vi "ReportOUT.vi"(0 "Full/Fails":string(combo)="Full", 1 "Operator":string, 2 "Original ATR Ref":refnum<vi>, 3 "GeneralResult":bool, 4 "Header Array":string[][](array[string]), 5 "error in (no error)":errorcluster, 6 "Header":string="                          Searcher EPC/Micro Card ATR", 7 "report file path":path, 8 "PN":string) -> (19 "error out":errorcluster)   [LabVIEW 2017]
uses:
  <vilib>/Utility/miscctls.llb/LVRowAndColumnUnsignedTypeDef.ctl
  <vilib>/Utility/NIReport.llb/Append Image to Report (path wrap).vi
  <vilib>/Utility/NIReport.llb/Append Text Table to Report (wrap).vi
  <vilib>/Utility/NIReport.llb/Append Report Text (str wrap).vi
  <vilib>/Utility/NIReport.llb/NI_report.lvclass
  <vilib>/Utility/NIReport.llb/Word/NI_Word.lvclass
  <vilib>/addons/_office/NI_ReportGenerationToolkit.lvlib
panel:
  in  "Pass  Button":bool
  in  "Fail  Button":bool
  in  "ATR To .docx":string[][](table)=array1670x7[11690 elements] caption="ATR"
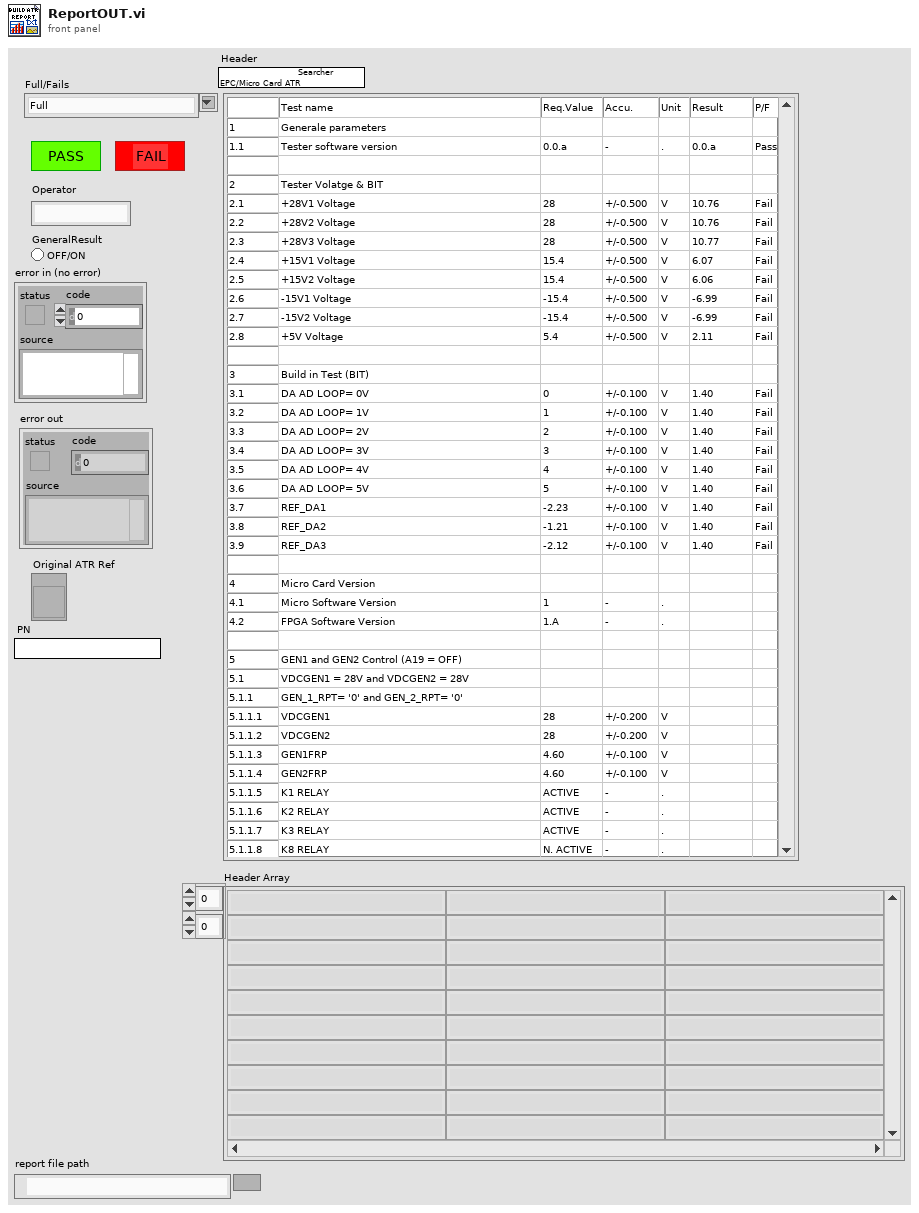
[diagram p1: front panel]
types:
  T1 = cluster{"top":dbl, "left":dbl, "right":dbl, "bottom":dbl}
  T2 = cluster{"alignment":enum16{"Left", "Centered", "Right", "Justify"}, "left":dbl, "right":dbl, "special":enum16{"(none)", "First line", "Hanging"}, "by":dbl, "before":dbl, "after":dbl, "line spacing":enum16{"Single", "1,5 lines", "Double", "At least", "Exactly", "Multiple"}, "at":dbl}
  T3 = enum16{"maximized", "minimized", "normal", "no change"}
  T4 = enum16{"Standard Report", "HTML", "Word", "Excel"}
  T5 = typedef "LVRowAndColumnUnsignedTypeDef.ctl" = cluster{"Row":u32, "Column":u32}
  T6 = typedef "LVFontTypeDef.ctl" = cluster{"Font Name":string, "Size":u16, "Bold":bool, "Italic":bool, "Underline":bool, "Strikeout":bool, "Color":u32}
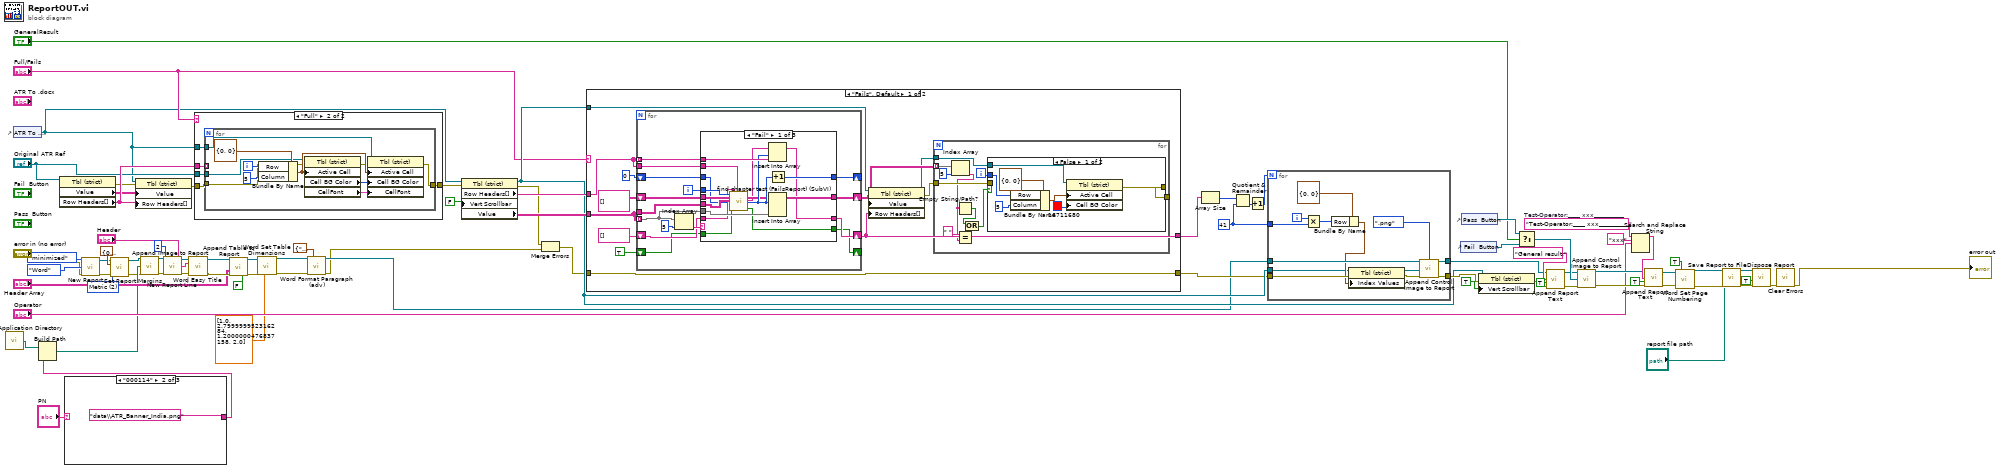
[diagram p0: block diagram]
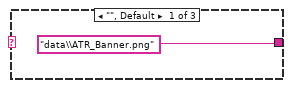
[diagram p2: hidden frame]
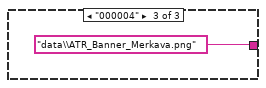
[diagram p3: hidden frame]
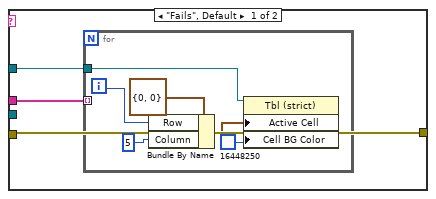
[diagram p4: hidden frame]
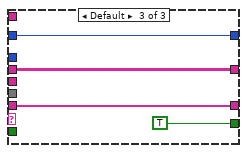
[diagram p7: hidden frame]
diagram:
  w7 = u16 2 items=["Default", "US", "Metric"] ("measurement system (default)")
  w64 = "Test-Operator:____ xxx__________"  # Test-Operator:____ xxx__________
  w77 = 41 ("y")
  n1 = call <vilib>:"Application Directory.vi"() -> ("Application Directory"=w14:path)
  n2 = control-ref of="ATR To .docx"() -> (w17:refnum<vi>)
  n3 = property class="Tbl (strict)"(reference="Original ATR Ref") -> (error out=w34:errorcluster, "Value"=w39:string[][], "Row Headers[]"=w40:string[])  [unwired: 1 in, 1 out]
  n4 = case shown="\"000114\"" "PN" {
    tunnel: ["data\\ATR_Banner.png" ("name or relative path") "data\\ATR_Banner_India.png" ("name or relative path") "data\\ATR_Banner_Merkava.png" ("name or relative path")] -> w13
    frame "", Default {
    }
    frame "000114" {
    }
    frame "000004" {
    }
  }
  n5 = Build Path(base path=w14, name or relative path=w13) -> (appended path=w8:path)
  n6 = call <vilib>:"New Report.vi"("window state (normal)"=T3."minimized", "report type"=T4."Word", "error in (no error)"="error in (no error)") -> ("report out"=w5:refnum<class "NI_report.lvclass">, "error out"=w4:errorcluster)  [unwired: 11 in]
  n7 = call-dynamic "Set Report Margins.vi"("report in"=w5, "margins (1.00)"=T1 {"top"=0.1, "left"=2.0, "right"=1.0, "bottom"=0.75}, "measurement system (default)"=w7, "error in (no error)"=w4) -> ("report out"=w2:refnum<class "NI_report.lvclass">, "error out"=w3:errorcluster)  [unwired: 9 in, 1 out]
  n8 = property class="Tbl (strict)"(reference=w17, error in=w34, "Value"=w39, "Row Headers[]"=w40) -> (error out=w67:errorcluster)  [unwired: 1 out]
  n9 = call-poly <vilib>:"Append Image to Report.vi"("report in"=w2, "path or URL of image"=w8, "error in (no error)"=w3) -> ("report out"=w10:refnum<class "NI_report.lvclass">, "error out"=w9:errorcluster)  [unwired: 9 in, 2 out]
  n10 = call-dynamic "New Report Line.vi"("report in"=w10, "number of lines (1)"=2, "error in (no error)"=w9) -> ("report out"=w23:refnum<class "NI_report.lvclass">, "error out"=w22:errorcluster)  [unwired: 11 in]
  n11 = call <vilib>:"Word Easy Title.vi"("report in"=w23, "title"="Header", "error in (no error)"=w22) -> ("report out"=w20:refnum<class "NI_report.lvclass">, "error out"=w21:errorcluster)  [unwired: 10 in, 1 out]
  n12 = case shown="\"Full\"" "Full/Fails" {
    tunnel: w17 -> [w85 w98]
    tunnel: "Original ATR Ref" -> [_ w97]
    tunnel: [w87 w96] -> w68
    tunnel: w67 -> [w87 w95]
    tunnel: w40 -> [w86 w94]
    frame "Fails", Default {
      n13 = for {
        tunnel: w86 -> [_] mode=indexing
        tunnel: w85 -> [w88]
        i -> [w93]
        n14 = Bundle By Name(cluster=T5 {"Row"=0, "Column"=0} ("Index Values"), "Row"=w93, "Column"=u32 5) -> (w91:T5)
        n15 = property class="Tbl (strict)"(reference=w88, "Active Cell"=w91, "Cell BG Color"=u32 16448250) -> ()  [unwired: 1 in, 2 out]
      }
    }
    frame "Full" {
      n16 = for {
        tunnel: w98 -> [w103]
        tunnel: w97 -> [w102]
        tunnel: [w101] -> w96
        tunnel: w95 -> [w99]
        tunnel: w94 -> [_] mode=indexing
        i -> [w104]
        n17 = Bundle By Name(cluster=T5 {"Row"=0, "Column"=0} ("Index Values"), "Row"=w104, "Column"=u32 5) -> (w106:T5)
        n18 = property class="Tbl (strict)"(reference=w102, error in=w99, "Active Cell"=w106) -> (error out=w100:errorcluster, "Cell BG Color"=w109:u32, "CellFont"=w108:T6)  [unwired: 1 out]
        n19 = property class="Tbl (strict)"(reference=w103, error in=w100, "Active Cell"=w106, "Cell BG Color"=w109, "CellFont"=w108) -> (error out=w101:errorcluster)  [unwired: 1 out]
      }
    }
  }
  n20 = call-poly <vilib>:"Append Table to Report.vi"("report in"=w20, "text data"="Header Array", "error in (no error)"=w21, "show grid lines (YES)"=FALSE) -> ("report out"=w48:refnum<class "NI_report.lvclass">, "error out"=w47:errorcluster)  [unwired: 8 in, 2 out]
  n21 = call <vilib>:"Word Set Table Dimensions.vi"("report in"=w48, "table column widths"=sgl[] [1.0, 2.8, 1.2, 2.0], "error in (no error)"=w47) -> ("report out"=w43:refnum<class "NI_report.lvclass">, "error out"=w42:errorcluster)  [unwired: 11 in]
  n22 = call <vilib>:"Word Format Paragraph (adv).vi"("report in"=w43, "indent and spacing"=T2 {"alignment"=enum."Left", "left"=0.0, "right"=0.0, "special"=enum."(none)", "by"=0.0, "before"=0.0, "after"=0.0, "line spacing"=enum."Single", "at"=0.0}, "error in (no error)"=w42) -> ("report out"=w41:refnum<class "NI_report.lvclass">, "error out"=w36:errorcluster)  [unwired: 11 in]
  n23 = property class="Tbl (strict)"(reference=w17, error in=w68, "Vert Scrollbar"=FALSE ("Visible Items:Vertical Scrollbar Visible")) -> (reference out=w70:refnum<vi>, error out=w37:errorcluster, "Row Headers[]"=w75:string[], "Value"=w74:string[][])
  n24 = Merge Errors(w37, w36) -> (w35:errorcluster)
  n25 = case shown="\"Fails\", Default" "Full/Fails" {
    tunnel: w35 -> [w121 w180]
    tunnel: w75 -> [w116 w181]
    tunnel: [w121 w180] -> w69
    tunnel: w74 -> [w117 _]
    tunnel: [w113 w181] -> w73
    tunnel: w70 -> [w114 _]
    frame "Fails", Default {
      n26 = for {
        tunnel: w117 -> [w149] mode=indexing
        shift-right: [w151] -> w112
        shift-left: string[][] [] -> [w153]
        shift-right: [w150] -> _
        shift-left: 0 -> [w152]
        tunnel: w116 -> [w147] mode=indexing
        shift-right: [w146] -> w113
        shift-left: string[] [] -> [w148]
        tunnel: w117 -> [w144]
        tunnel: w116 -> [w143]
        shift-right: [w141] -> _
        shift-left: TRUE -> [w142]
        i -> [w145]
        n27 = Index Array(array=w149, index=5) -> (element=w154:string)
        n28 = case shown="\"Fail\"" w154 {
          tunnel: w153 -> [w165 w174 w178]
          tunnel: w152 -> [w162 w175 w179]
          tunnel: [w171 w174 w178] -> w151
          tunnel: [w170 w175 w179] -> w150
          tunnel: w149 -> [w169 _ _]
          tunnel: w148 -> [w164 w173 w177]
          tunnel: w147 -> [w163 _ _]
          tunnel: [w168 w173 w177] -> w146
          tunnel: w145 -> [w166 _ _]
          tunnel: w144 -> [w167 _ _]
          tunnel: w143 -> [w158 _ _]
          tunnel: w142 -> [w157 w172 _]
          tunnel: [w156 w172 TRUE ("ToExecute? Out")] -> w141
          frame "Fail" {
            n29 = call "find chapter test (FailsReport) (SubVI).vi"("ForLoopIndex"=w166, "Fails ATR IN"=w165, "Full ATR"=w167, "FailsATR Index IN"=w162, "ToExecute?"=w157, "Fails ATR RowHeader IN"=w164, "Full ATR RowHeader"=w158) -> ("Fails ATR OUT"=w160:string[][], "Fails ATR RowHeader OUT"=w159:string[], "FailsATR Index OUT"=w161:i32, "ToExecute? Out"=w156:bool)  [unwired: 9 in]
            n30 = Insert Into Array(array=w159, index=w161, new element=w163) -> (w168:string[])
            n31 = Insert Into Array(array=w160, index (row)=w161, new element=w169) -> (w171:string[][])  [unwired: 1 in]
            n32 = Increment(x=w161) -> (x+1=w170:i32)
          }
          frame "Pass" {
          }
          frame Default {
          }
        }
      }
      n33 = property class="Tbl (strict)"(reference=w114, "Value"=w112, "Row Headers[]"=w113) -> (reference out=w110:refnum<vi>, error out=w111:errorcluster)  [unwired: 1 in]
      n34 = for {
        tunnel: [w131] -> _
        tunnel: w112 -> [w130] mode=indexing
        tunnel: w111 -> [w128]
        tunnel: w110 -> [w127]
        i -> [w132]
        n35 = Index Array(array=w130, index=5) -> (element=w124:string)
        n36 = Empty String/Path?(string/path=w124) -> (empty?=w126:bool)
        n37 = Equal?(x=" ", y=w124) -> (x = y?=w123:bool)
        n38 = Or(x=w126, y=w123) -> (x .or. y?=w122:bool)
        n39 = case shown="False" w122 {
          tunnel: w132 -> [w136 _]
          tunnel: [w135 w140] -> w131
          tunnel: w128 -> [_ w140]
          tunnel: w127 -> [w133 _]
          frame False {
            n40 = Bundle By Name(cluster=T5 {"Row"=0, "Column"=0} ("Index Values"), "Row"=w136, "Column"=u32 5) -> (w138:T5)
            n41 = property class="Tbl (strict)"(reference=w133, "Active Cell"=w138, "Cell BG Color"=u32 16711680) -> (error out=w135:errorcluster)  [unwired: 1 in, 1 out]
          }
          frame True {
          }
        }
      }
    }
    frame "Full" {
    }
  }
  n42 = Array Size(array=w73) -> (size(s)=w78:i32)
  n43 = Quotient & Remainder(x=w78, y=w77) -> (floor(x/y)=w79:i32)  [unwired: 1 out]
  n44 = Increment(x=w79) -> (x+1=w80:i32)
  n45 = for {
    N: w80 -> [_]
    tunnel: w77 -> [w191]
    tunnel: w41 -> [w189]
    tunnel: w69 -> [w186]
    tunnel: [w188] -> w71
    tunnel: w70 -> [w183]
    tunnel: [w182] -> w58
    i -> [w192]
    n46 = Multiply(x=w192, y=w191) -> (x*y=w193:i32)
    n47 = Bundle By Name(cluster=T5 {"Row"=0, "Column"=0} ("Index Values"), "Row"=w193) -> (w185:T5)
    n48 = property class="Tbl (strict)"(reference=w183, error in=w186, "Index Values"=w185) -> (reference out=w184:refnum<vi>, error out=w187:errorcluster)
    n49 = call-dynamic "Append Control Image to Report.vi"("report in"=w189, "image file type (.jpg)"=enum16{".jpg", ".png"}.".png" ("image file type(.jpg)"), "ctrl reference"=w184, "error in (no error)"=w187) -> ("report out"=w182:refnum<class "NI_report.lvclass">, "error out"=w188:errorcluster)  [unwired: 8 in, 2 out]
  }
  n50 = control-ref of="Fail  Button"() -> (w60:refnum<vi>)
  n51 = control-ref of="Pass  Button"() -> (w61:refnum<vi>)
  n52 = property class="Tbl (strict)"(reference=w70, error in=w71, "Vert Scrollbar"=TRUE ("Visible Items:Vertical Scrollbar Visible")) -> (error out=w56:errorcluster)  [unwired: 1 out]
  n53 = Select(t=w61, s="GeneralResult", f=w60) -> (s? t:f=w62:refnum<vi>)
  n54 = call-poly <vilib>:"Append Report Text.vi"("report in"=w58, "text"="General result:", "append on new line? (F)"=TRUE, "error in (no error)"=w56) -> ("report out"=w54:refnum<class "NI_report.lvclass">, "error out"=w55:errorcluster)  [unwired: 8 in, 2 out]
  n55 = call-dynamic "Append Control Image to Report.vi"("report in"=w54, "ctrl reference"=w62, "error in (no error)"=w55) -> ("report out"=w53:refnum<class "NI_report.lvclass">, "error out"=w52:errorcluster)  [unwired: 9 in, 2 out]
  n56 = Search and Replace String(input string=w64, search string="xxx", replace string="Operator") -> (result string=w63:string)  [unwired: 5 in, 3 out]
  n57 = call-poly <vilib>:"Append Report Text.vi"("report in"=w53, "text"=w63, "append on new line? (F)"=TRUE, "error in (no error)"=w52) -> ("report out"=w31:refnum<class "NI_report.lvclass">, "error out"=w30:errorcluster)  [unwired: 8 in, 2 out]
  n58 = call <vilib>:"Word Set Page Numbering.vi"("report in"=w31, "include page x of n"=TRUE, "error in (no error)"=w30) -> ("report out"=w28:refnum<class "NI_report.lvclass">, "error out"=w29:errorcluster)  [unwired: 11 in]
  n59 = call-dynamic "Save Report to File.vi"("report in"=w28, "report file path"="report file path", "error in (no error)"=w29) -> ("report out"=w26:refnum<class "NI_report.lvclass">, "error out"=w27:errorcluster)  [unwired: 11 in]
  n60 = call-dynamic "Dispose Report.vi"("report in"=w26, "save changes? (F)"=TRUE, "error in (no error)"=w27) -> ("error out"=w16:errorcluster)  [unwired: 12 in]
  n61 = call <vilib>:"Clear Errors.vi"("error in (no error)"=w16) -> ("error out"=→"error out":errorcluster)  [unwired: 5 in, 1 out]
